vi "Do.vi"(8 "error in (no error)":errorcluster, 10 "Actor in":refnum<class "Actor.lvclass">, 11 "Data Generator Msg":refnum<class "Data Generator Msg.lvclass">) -> (0 "error out":errorcluster, 2 "Actor out":refnum<class "Actor.lvclass">)   [LabVIEW 2015, in "Data Generator Msg.lvclass"]
doc: "This VI delivers the message to the actor by calling the appropriate method(s) on the actor."
uses:
  Data Generator Msg.lvclass
  Zen Analytics/Zen Analytics.lvclass
  <vilib>/ActorFramework/Actor/Actor.lvclass
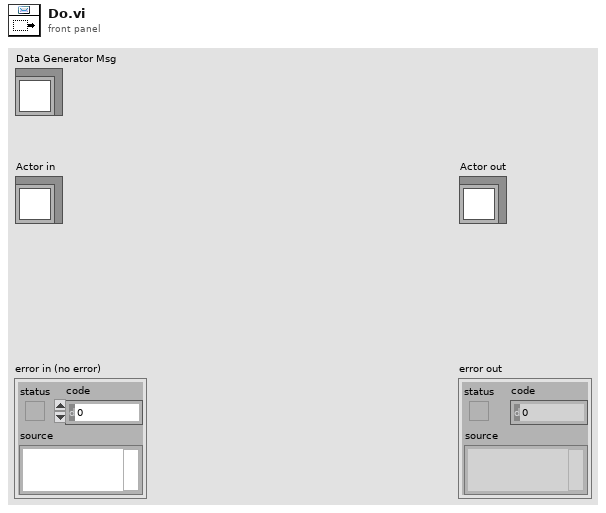
[diagram p1: front panel]
types:
  T1 = cluster{"InitializationParams":cluster{"CurrentPartNumber":string, "MeasurementData":cluster{"MeasurementID":i32, "MeasureEnable":bool, "MeasurementPass":bool, "LimitSets":cluster{"LimitSetId":i32, "Limits":dbl[]}[]}[]}}
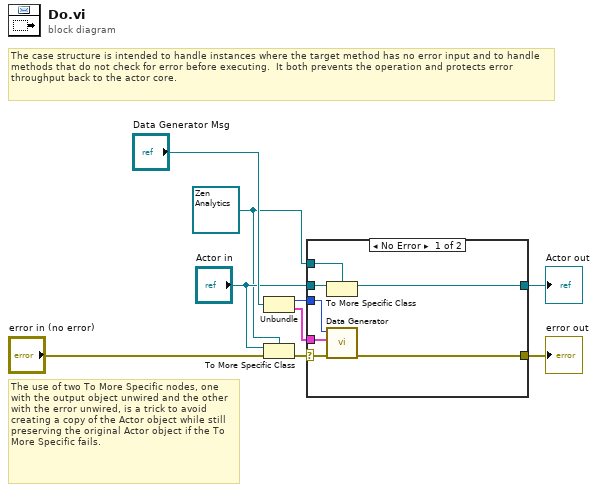
[diagram p0: block diagram]
diagram:
  w3 = refnum<class "Zen Analytics.lvclass"> refnum ("Actor in")
  # "The use of two To More Specific nodes, one with the output object unwired and the other with the error unwired, is a trick to avoid creating a copy of the Actor object while still preserving the original Actor object if the To More Specific fails."
  # "The case structure is intended to handle instances where the target method has no error input and to handle methods that do not check for error before executing.  It both prevents the operation and protects error throughput back to the actor core."
  n1 = Unbundle("Data Generator Msg") -> (w2:u32, w1:T1)
  n2 = To More Specific Class(target class=w3, reference="Actor in", error in="error in (no error)") -> (error out=w7:errorcluster)  [unwired: 1 out]
  n3 = case shown="No Error" w7 {
    selector: w7 -> [w15 w18]
    tunnel: [w16 w18] -> w6
    tunnel: [w12 w17] -> w5
    tunnel: "Actor in" -> [w14 w17]
    tunnel: w3 -> [w13 _]
    tunnel: w2 -> [w11 _]
    tunnel: w1 -> [w10 _]
    frame No Error {
      n4 = To More Specific Class(target class=w13, reference=w14) -> (specific class reference=w12:refnum<class "Zen Analytics.lvclass">)  [unwired: 1 in, 1 out]
      n5 = call "Data Generator.vi"("error in"=w15, "Initialization Values"=w10, "I"=w11) -> ("error out"=w16:errorcluster)  [unwired: 4 in, 4 out]
    }
    frame Error {
      # "If type check fails, pass the original object out again."
    }
  }
  "error out" <- w6
  "Actor out" <- w5
